vi "gate open-close.vi"(8 "error in (no error)":errorcluster, 11 "button value":bool) -> (0 "error out":errorcluster)   [LabVIEW 2014]
uses:
  <vilib>/Rock Robotics/WPI/Solenoid/WPI_SolenoidValue.ctl
  <vilib>/Rock Robotics/WPI/Solenoid/Deprecated/WPI_SolenoidGetBool.vi
  <vilib>/Rock Robotics/WPI/Solenoid/WPI_SolenoidSetEnum.vi
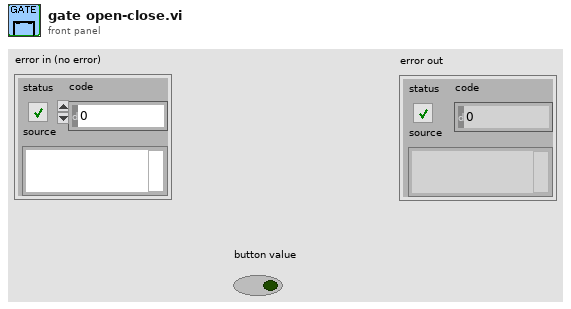
[diagram p1: front panel]
types:
  T1 = typedef "WPI_SolenoidValue.ctl" = enum16{"Off", "On", "Forward", "Reverse"}
  T2 = typedef "WPI_SolenoidDevRef.ctl" = cluster{"DevStatus":errorcluster, "Pneumatics Control Module":u8, "Forward Solenoid Channel":T3, "Reverse Solenoid Channel":T3}
  T3 = typedef "WPI_SolenoidChannel.ctl" = enum8{"Solenoid 0", "Solenoid 1", "Solenoid 2", "Solenoid 3", "Solenoid 4", "Solenoid 5", "Solenoid 6", "Solenoid 7", "Invalid"}
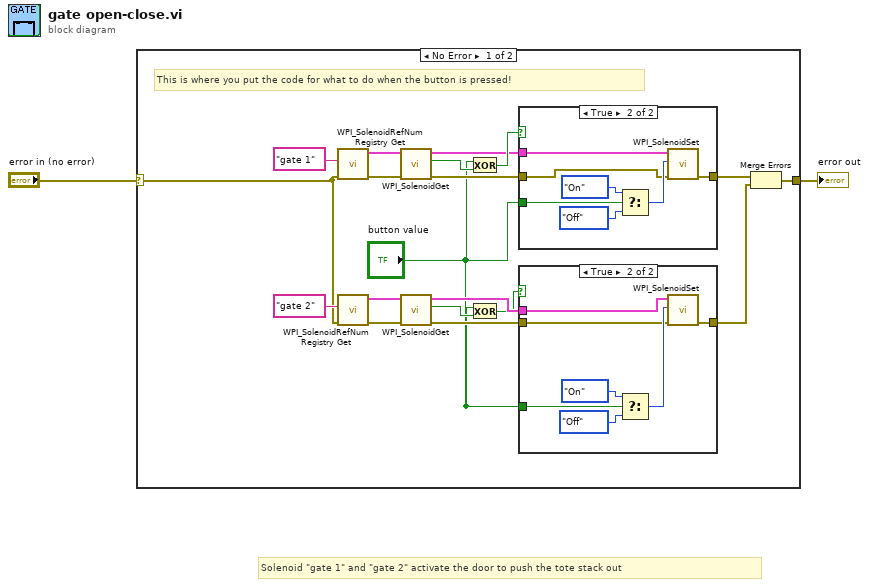
[diagram p0: block diagram]
diagram:
  # "Solenoid \"gate 1\" and \"gate 2\" activate the door to push the tote stack out"
  n1 = case shown="No Error" "error in (no error)" {
    selector: "error in (no error)" -> [w7 w38]
    tunnel: [w4 w38] -> w1
    frame No Error {
      # "This is where you put the code for what to do when the button is pressed!"
      n2 = call <vilib>:"WPI_SolenoidRefNum Registry Get.vi"("error in (no error)"=w7, "refnum name"="gate 1") -> ("error out"=w16:errorcluster, "SolenoidDevRef"=w19:T2)  [unwired: 8 in]
      n3 = call <vilib>:"WPI_SolenoidRefNum Registry Get.vi"("error in (no error)"=w7, "refnum name"="gate 2") -> ("error out"=w13:errorcluster, "SolenoidDevRef"=w10:T2)  [unwired: 8 in]
      n4 = call-poly <vilib>:"WPI_SolenoidGet.vi"("error in (no error)"=w16, "SolenoidDevRef"=w19) -> ("error out"=w15:errorcluster, "Value"=w21:bool, "SolenoidDevRef"=w18:T2)  [unwired: 7 in]
      n5 = call-poly <vilib>:"WPI_SolenoidGet.vi"("error in (no error)"=w13, "SolenoidDevRef"=w10) -> ("error out"=w14:errorcluster, "Value"=w8:bool, "SolenoidDevRef"=w11:T2)  [unwired: 7 in]
      n6 = Exclusive Or(1:w21, 2:"button value") -> (0:w20:bool)
      n7 = Exclusive Or(1:w8, 2:"button value") -> (0:w9:bool)
      n8 = case shown="True" w20 {
        tunnel: w18 -> [_ w37]
        tunnel: "button value" -> [_ w36]
        tunnel: w15 -> [w30 w32]
        tunnel: [w30 w31] -> w5
        frame False {
        }
        frame True {
          n9 = Select(t=WPI_SolenoidValue."On" ("Value"), s=w36, f=WPI_SolenoidValue."Off" ("Value")) -> (s? t:f=w33:T1)
          n10 = call-poly <vilib>:"WPI_SolenoidSet.vi"("error in (no error)"=w32, "Value"=w33, "SolenoidDevRef"=w37) -> ("error out"=w31:errorcluster)  [unwired: 7 in, 1 out]
        }
      }
      n11 = case shown="True" w9 {
        tunnel: w11 -> [_ w29]
        tunnel: "button value" -> [_ w28]
        tunnel: w14 -> [w22 w24]
        tunnel: [w22 w23] -> w6
        frame False {
        }
        frame True {
          n12 = Select(t=WPI_SolenoidValue."On" ("Value"), s=w28, f=WPI_SolenoidValue."Off" ("Value")) -> (s? t:f=w25:T1)
          n13 = call-poly <vilib>:"WPI_SolenoidSet.vi"("error in (no error)"=w24, "Value"=w25, "SolenoidDevRef"=w29) -> ("error out"=w23:errorcluster)  [unwired: 7 in, 1 out]
        }
      }
      n14 = Merge Errors(w5, w6) -> (w4:errorcluster)
    }
    frame Error {
      # "This is what to do if there is an error.  Usually it is nothing."
    }
  }
  "error out" <- w1
